vi "Coefficients to String.vi"(11 "IIR Filter Cluster":T1) -> (3 "String":string)   [LabVIEW 2019, in "DSP.lvclass"]
uses:
  DSP.lvclass
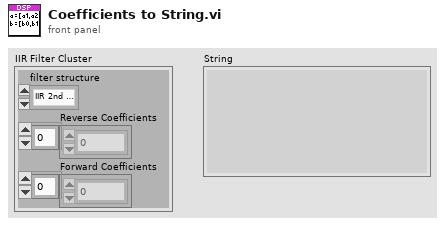
[diagram p1: front panel]
types:
  T1 = cluster{"filter structure":enum32{"IIR 2nd Order", "IIR 4th Order"}, "Reverse Coefficients":dbl[], "Forward Coefficients":dbl[]}
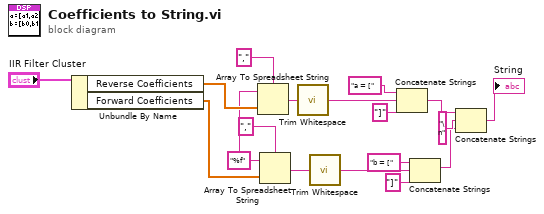
[diagram p0: block diagram]
diagram:
  w9 = "%f" ("format string")
  n1 = Unbundle By Name("IIR Filter Cluster") -> ("Reverse Coefficients"=w18:dbl[], "Forward Coefficients"=w17:dbl[])
  n2 = Array To Spreadsheet String(delimiter (Tab)=",", array=w18, 3:w9) -> (spreadsheet string=w3:string)
  n3 = Array To Spreadsheet String(delimiter (Tab)=",", array=w17, 3:w9) -> (spreadsheet string=w8:string)
  n4 = call <vilib>:"Trim Whitespace.vi"("string"=w3) -> ("trimmed string"=w14:string)  [unwired: 1 in]
  n5 = call <vilib>:"Trim Whitespace.vi"("string"=w8) -> ("trimmed string"=w15:string)  [unwired: 1 in]
  n6 = Concatenate Strings("a = [" ("string"), w14, "]" ("string")) -> (w10:string)
  n7 = Concatenate Strings("b = [" ("string"), w15, "]" ("string")) -> (w11:string)
  n8 = Concatenate Strings(w10, "\n" ("string"), w11) -> (→"String":string)
